vi "SPIEngineSOM.vi"(7 "NumNodes":u8=4) -> (2 "Out Vld":u8, 3 "Cmd Rcv":u8)   [LabVIEW 2014, in "IO Node Logic Template_SPIBus0.lvlib"]
uses:
  IO Node Logic Template_SPIBus0.lvlib
  <userlib>/_NI SPI IP/FPGA/Controllers/Public/Spi Master Outputs.ctl
  <vilib>/SPIAPI/DIO/SPI DIO Enable Lines.ctl
  Controls/All Nodes Resources.ctl
  Node/Controls/NodeResources FIFOs.ctl
  <vilib>/SPIAPI/DIO/SPI Digital IO Lines.ctl
  <vilib>/Platform/TimedLoop/XDataNode/timing_clust.ctl
  <vilib>/Platform/TimedLoop/XDataNode/nitl_modes.ctl
  <vilib>/Platform/TimedLoop/XDataNode/wakeup.ctl
  <vilib>/rvi/Emulation/niFpgaSctlEmulationGetInTimedLoop.vi
  <vilib>/rvi/Emulation/niFpgaEmulationReportErrorSimple.vi
  <vilib>/rvi/Emulation/niFpgaGetClockAttributes.vi
  <vilib>/rvi/Emulation/niFpgaCriticalErrorInLSC.vi
  <instrlib>/_niInstr/Basic Elements/v1/FPGA/Private/Count Up U8.vi
  <vilib>/Platform/TimedLoop/XDataNode/XDataNode.xnode
  <vilib>/Platform/TimedLoop/XDataNode/XDNodeRunTimeDep.lvlib
  <instrlib>/_niInstr/Basic Elements/v1/FPGA/niInstr Basic Elements v1 FPGA.lvlib
  <userlib>/_NI SPI IP/FPGA/Controllers/NI SPI IP FPGA.lvlib
panel:
  out "spi output":T1
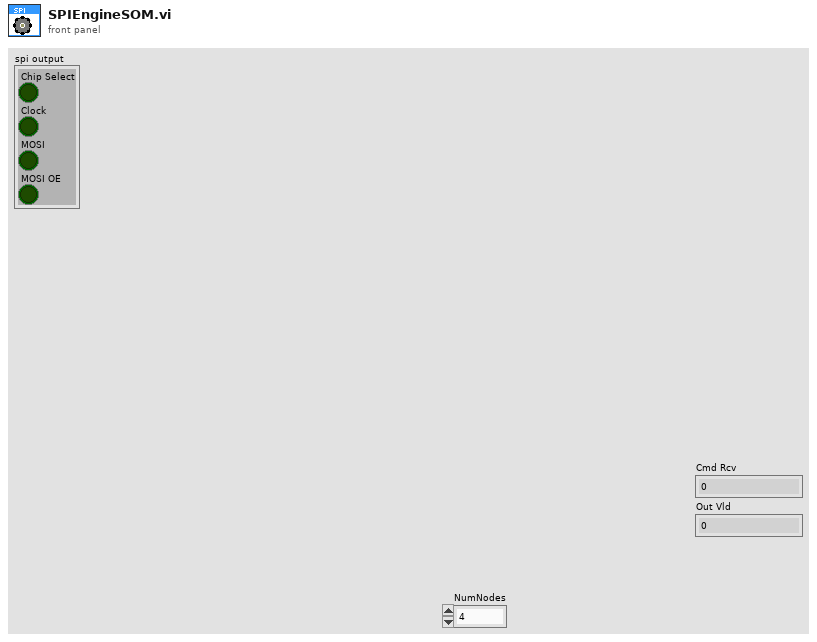
[diagram p1: front panel]
types:
  T1 = typedef "NI SPI IP FPGA.lvlib/Spi Master Outputs.ctl" = cluster{"Chip Select":bool, "Clock":bool, "MOSI":bool, "MOSI OE":bool}
  T2 = typedef "SPI Digital IO Lines.ctl" = cluster{"SCLK":refnum<k21>, "MISO":refnum<k21>, "MOSI":refnum<k21>, "CS 0":refnum<k21>, "CS 1":refnum<k21>, "CS 2":refnum<k21>, "CS 3":refnum<k21>, "CS 4":refnum<k21>, "CS 5":refnum<k21>}
  T3 = typedef "IO Node Logic Template_SPIBus0.lvlib/All Nodes Resources.ctl" = cluster{"FIFOs.Node 0":T4, "FIFOs.Node 1":T4, "FIFOs.Node 2":T4, "FIFOs.Node 3":T4}
  T4 = typedef "IO Node Logic Template_SPIBus0.lvlib/NodeResources FIFOs.ctl" = cluster{"SendCmdFIFO":refnum<k21>, "ReceiveDataFIFO":refnum<k21>}
  T5 = typedef "SPI DIO Enable Lines.ctl" = cluster{"SCLK_en":refnum<k21>, "MISO_en":refnum<k21>, "MOSI_en":refnum<k21>, "CS0_en":refnum<k21>, "CS1_en":refnum<k21>, "CS2_en":refnum<k21>, "CS3_en":refnum<k21>, "CS4_en":refnum<k21>, "CS5_en":refnum<k21>}
  T6 = typedef "Internal Data (SPI API).ctl" = cluster{"DLU To SPI Engine Data FIFO":refnum<k21>, "SPI Engine to DLU Data FIFO":refnum<k21>, "Data to SPI Engine (Cache) Register":refnum<k21>, "SPI PHY Settings to SPI Engine (Cahche) Register":refnum<k21>}
  T7 = typedef "XDNodeRunTimeDep.lvlib/timing_clust.ctl" = cluster{"Expected End [f-1]":u64, "Actual End [f-1]":u64, "Finished Late? [f-1]":bool, "Expected End [i-1]":u64, "Actual End [i-1]":u64, "Finished Late? [i-1]":bool, "Expected Start [i]":u64, "Actual Start [i]":u64, "Expected Start [f]":u64, "Actual Start [f]":u64, "Source Name":string, "Structure Name":string, "Period":i64, "Deadline":i64, "Offset":i64, "Start":i64, "Priority":i32, "Timeout":i32, "Mode":T8, "Wakeup Reason":T9, "Error":errorcluster, "Source Type":string, "Secondary Source Type":string, "Global End Time":u64, "Global Start Time":u64, "Frame Duration":u64, "Iteration Duration":u64, "Assigned CPU":i32, "I/O Scan Engine Mode":u32}
  T8 = typedef "XDNodeRunTimeDep.lvlib/nitl_modes.ctl" = enum32{"No Change", "Process missed periods, maintain original phase", "Discard missed periods, maintain original phase", "Process missed periods, ignore original phase", "Discard missed periods, ignore original phase"}
  T9 = typedef "XDNodeRunTimeDep.lvlib/wakeup.ctl" = enum32{"Normal", "Aborted", "Asynchronous wakeup", "Timing source error", "Timed loop error", "Timeout"}
  T10 = typedef "IO Node Logic Template_SPIBus0.lvlib/Node_Command_Sent.ctl" = cluster{"Device ID":u8, "Data":u64, "Command":u8, "Node ID":u8, "Misc":u8}
  T11 = typedef "SPI Response Information.ctl" = cluster{"Data to Node":u64, "Node Id":u16}
  T12 = typedef "NI SPI IP FPGA.lvlib/Spi Master Inputs.ctl" = cluster{"MISO":bool}
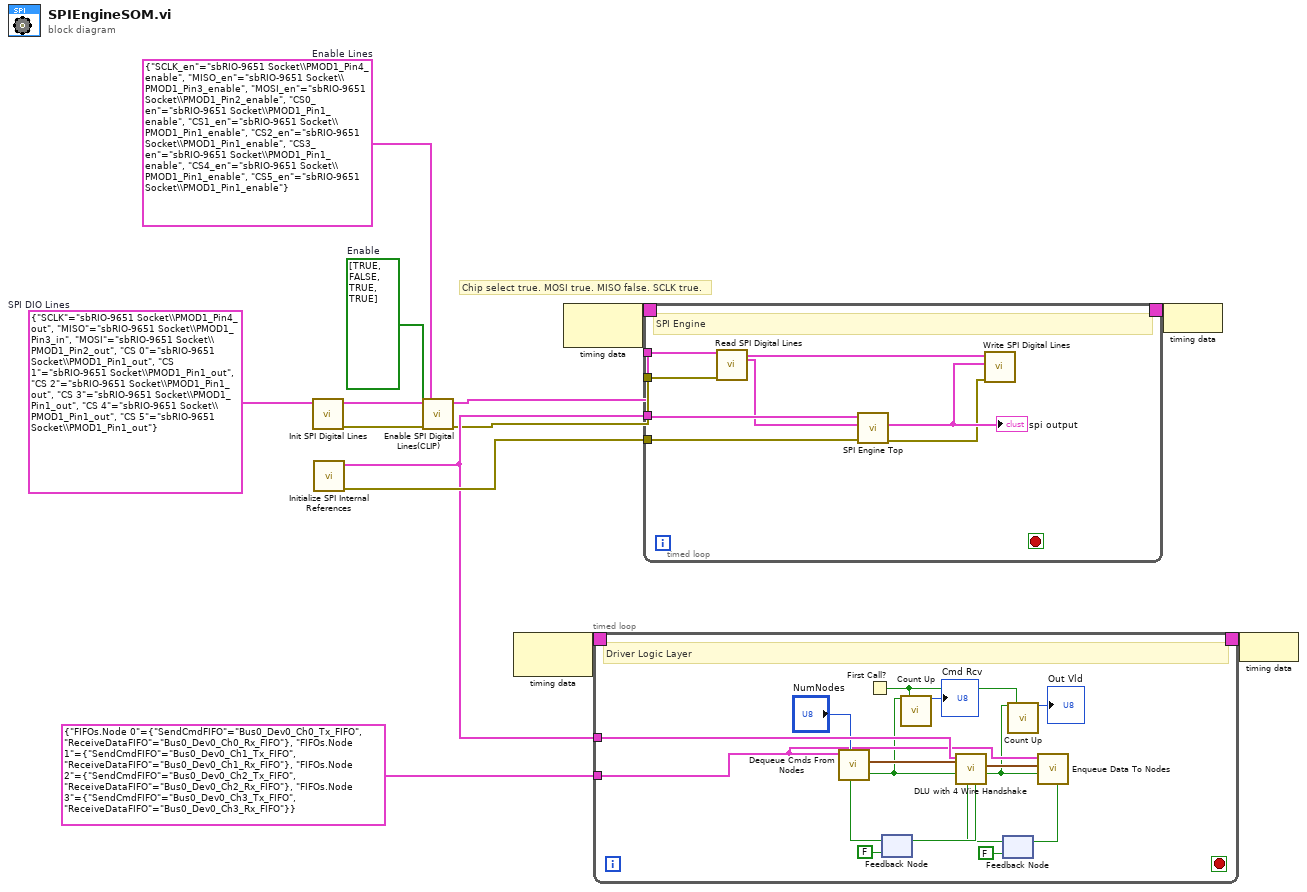
[diagram p0: block diagram]
diagram:
  w8 = T2 {"SCLK"="sbRIO-9651 Socket\\PMOD1_Pin4_out", "MISO"="sbRIO-9651 Socket\\PMOD1_Pin3_in", "MOSI"="sbRIO-9651 Socket\\PMOD1_Pin2_out", "CS 0"="sbRIO-9651 Socket\\PMOD1_Pin1_out", "CS 1"="sbRIO-9651 Socket\\PMOD1_Pin1_out", "CS 2"="sbRIO-9651 Socket\\PMOD1_Pin1_out", "CS 3"="sbRIO-9651 Socket\\PMOD1_Pin1_out", "CS 4"="sbRIO-9651 Socket\\PMOD1_Pin1_out", "CS 5"="sbRIO-9651 Socket\\PMOD1_Pin1_out"}  # SPI DIO Lines
  w4 = bool[] [TRUE, FALSE, TRUE, TRUE]  # Enable
  w5 = T5 {"SCLK_en"="sbRIO-9651 Socket\\PMOD1_Pin4_enable", "MISO_en"="sbRIO-9651 Socket\\PMOD1_Pin3_enable", "MOSI_en"="sbRIO-9651 Socket\\PMOD1_Pin2_enable", "CS0_en"="sbRIO-9651 Socket\\PMOD1_Pin1_enable", "CS1_en"="sbRIO-9651 Socket\\PMOD1_Pin1_enable", "CS2_en"="sbRIO-9651 Socket\\PMOD1_Pin1_enable", "CS3_en"="sbRIO-9651 Socket\\PMOD1_Pin1_enable", "CS4_en"="sbRIO-9651 Socket\\PMOD1_Pin1_enable", "CS5_en"="sbRIO-9651 Socket\\PMOD1_Pin1_enable"}  # Enable Lines
  # "Chip select true. MOSI true. MISO false. SCLK true."
  n1 = call <vilib>:"Init SPI Digital Lines.vi"("Chip Select DIO Lines"=w8) -> ("error out"=w3:errorcluster, "Chip Select DIO Lines"=w6:T2)  [unwired: 9 in]
  n2 = call <vilib>:"Initialize SPI Internal References.vi"() -> ("error out"=w14:errorcluster, "SPI API References"=w13:T6)  [unwired: 10 in]
  n3 = call <vilib>:"Enable SPI Digital Lines(CLIP).vi"("error in"=w3, "Enable"=w4, "Enable Lines"=w5, "SPI DIO Lines"=w6) -> ("error out"=w2:errorcluster, "Chip Select DIO Lines"=w1:T2)  [unwired: 6 in]
  n4 = node-c288() -> (w10:T7)  [unwired: 1 in]
  n5 = node-c288() -> (w12:T7)  [unwired: 1 in]
  n6 = timed-loop {
    tunnel: w13 -> [w23]
    timing: w10 -> [_]
    timing-out: [_] -> w9
    tunnel: T3 {"FIFOs.Node 0"={"SendCmdFIFO"="Bus0_Dev0_Ch0_Tx_FIFO", "ReceiveDataFIFO"="Bus0_Dev0_Ch0_Rx_FIFO"}, "FIFOs.Node 1"={"SendCmdFIFO"="Bus0_Dev0_Ch1_Tx_FIFO", "ReceiveDataFIFO"="Bus0_Dev0_Ch1_Rx_FIFO"}, "FIFOs.Node 2"={"SendCmdFIFO"="Bus0_Dev0_Ch2_Tx_FIFO", "ReceiveDataFIFO"="Bus0_Dev0_Ch2_Rx_FIFO"}, "FIFOs.Node 3"={"SendCmdFIFO"="Bus0_Dev0_Ch3_Tx_FIFO", "ReceiveDataFIFO"="Bus0_Dev0_Ch3_Rx_FIFO"}} ("Communication FIFOs") -> [w20]
    stop <- _ stop-if-true
    # "Driver Logic Layer"
    n7 = First Call?() -> (First Call?: T/F=w17:bool)
    n8 = feedback #1(FALSE ("Ready For Input?")) -> (w29:bool)
    n9 = call "Dequeue Cmds From Nodes.vi"("Ready For Output?"=w29, "NumNodes"="NumNodes", "Communication FIFOs"=w20) -> ("Cmd Received Valid"=w18:bool, "Cmd Received"=w27:T10)  [unwired: 5 in, 2 out]
    n10 = call-poly <instrlib>:"Count Up.vi"("increment"=w18, "reset"=w17) -> ("count out"=→"Cmd Rcv":u8)  [unwired: 13 in]
    n11 = feedback #2(FALSE ("Ready for Input")) -> (w25:bool)
    n12 = call "DLU with 4 Wire Handshake.vi"("ready for output"=w25, "Input Valid"=w18, "Input Data"=w27, "Private Data In"=w23) -> ("Output Valid"=w19:bool, "Output Data"=w22:T11, "ready for Input"=w28:bool)  [unwired: 5 in]
    n13 = feedback-in #1(w28) -> ()
    n14 = call-poly <instrlib>:"Count Up.vi"("increment"=w19, "reset"=w17) -> ("count out"=→"Out Vld":u8)  [unwired: 13 in]
    n15 = call "Enqueue Data To Nodes.vi"("Input Valid"=w19, "Input Data"=w22, "Communication FIFOs"=w20) -> ("Ready for Input"=w26:bool)  [unwired: 6 in, 2 out]
    n16 = feedback-in #2(w26) -> ()
  }
  n17 = timed-loop {
    tunnel: w13 -> [w40]
    tunnel: w14 -> [w39]
    tunnel: w1 -> [w38]
    tunnel: w2 -> [w37]
    timing: w12 -> [_]
    timing-out: [_] -> w11
    stop <- _ stop-if-true
    # "SPI Engine"
    n18 = call <vilib>:"Read SPI Digital Lines.vi"("Chip Select DIO Lines"=w38, "error in"=w37) -> ("Chip Select DIO Lines Out"=w36:T2, "SPI Read Data"=w34:T12)  [unwired: 11 in, 1 out]
    n19 = call <vilib>:"SPI Engine Top.vi"("error in"=w39, "SPI Read Data"=w34, "SPI API References"=w40) -> ("error out"=w33:errorcluster, "SPI DIO Output"=w35:T1)  [unwired: 5 in, 2 out]
    "spi output" <- w35
    n20 = call <vilib>:"Write SPI Digital Lines.vi"("error in"=w33, "spi output"=w35, "Chip Select DIO Lines"=w36) -> ()  [unwired: 7 in, 2 out]
  }
  n21 = node-c288(w11) -> ()
  n22 = node-c288(w9) -> ()
